vi "POLARIS Image Viewer.vi"() -> ()   [LabVIEW 2014]
uses:
  XDisplay/POLARIS IMAQ Display.xctl
  XDisplay/Properties/ImageSource.ctl
  Analyze Classes/Analyze BaseClass/Analyze BaseClass.lvclass
  Utility/POLARIS Vision utility.lvlib
panel:
  out "error out":errorcluster
  in  "File":path=path "D:/Test XDisplay images/Test TargetFocus/Test Report REad_A4 q=0,00  A=Inf µm2 _JustageCam 201410-30 16.08.30 - Kopie.png"
  out "XDisplay":cluster{"Image":T1}(xcontrol)={"Image"="remote image 000000000D10E76C"}
  in  "stop":bool=TRUE
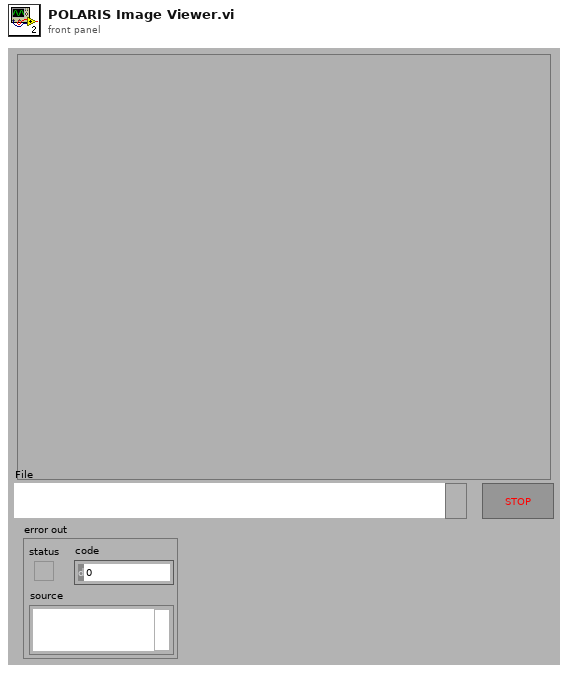
[diagram p1: front panel]
types:
  T1 = typedef "IMAQ Image.ctl" = refnum<image>
  T2 = typedef "POLARIS IMAQ Display.xctl/ImageSource.ctl" = enum16{"Camera", "File"}
  T3 = typedef "Image Type" = u32
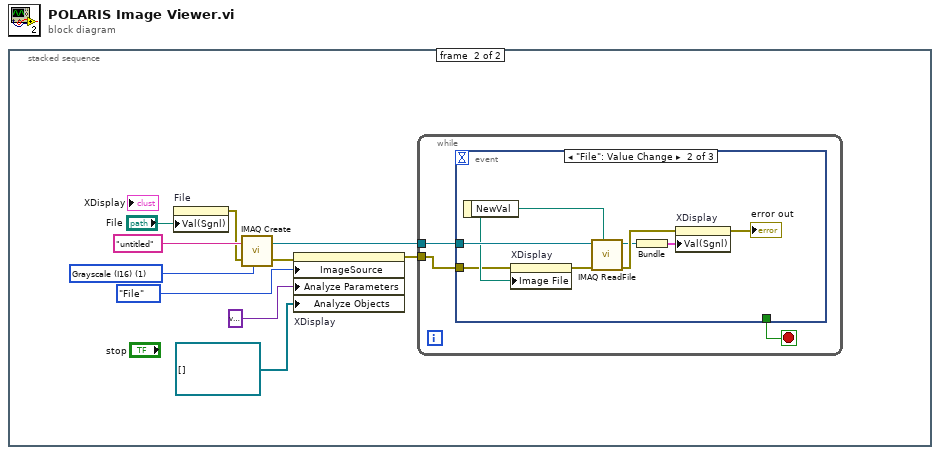
[diagram p0: block diagram]
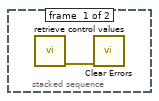
[diagram p2: hidden frame]
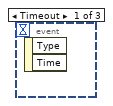
[diagram p3: hidden frame]
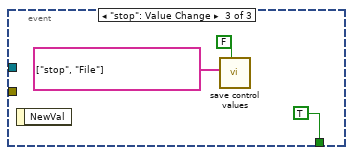
[diagram p4: hidden frame]
diagram:
  n1 = stacked-sequence {
    frame #0 {
      n2 = call "retrieve control values.vi"() -> ("error out"=w1:errorcluster)  [unwired: 10 in, 1 out]
      n3 = call <vilib>:"Clear Errors.vi"("error in (no error)"=w1) -> ()  [unwired: 5 in, 2 out]
    }
    frame #1 {
      w7 = T3 1 items=["Grayscale (U8)", "Grayscale (I16)", "Grayscale (SGL)", "Complex (CSG)", "RGB (U32)", "HSL (U32)", "RGB (U64)", "Grayscale (U16)"] ("Image Type")
      n4 = property on="File" class="Path"("Val(Sgnl)"="File") -> (error out=w4:errorcluster)  [unwired: 2 in, 1 out]
      n5 = call "IMAQ Create"("Image Name"="untitled", "Image Type"=w7, "error in (no error)"=w4) -> ("New Image"=w10:T1, "error out"=w9:errorcluster)  [unwired: 2 in]
      n6 = property on="XDisplay" class="POLARIS IMAQ Display (strict)"(error in=w9, "ImageSource"=ImageSource."File", "Analyze Parameters"=variant, "Analyze Objects"=refnum<class "Analyze BaseClass.lvclass">[] []) -> (error out=w6:errorcluster)  [unwired: 1 in, 1 out]
      n7 = while {
        tunnel: w6 -> [w12]
        tunnel: w10 -> [w13]
        stop <- w14 stop-if-true
        n8 = event shown="[1] \"File\": Value Change" {
          selector: _ -> [_ _ _]
          dyn-events: _ -> [_ _ _]
          timeout: _ -> [_ _ _]
          tunnel: [_ _ TRUE] -> w14
          tunnel: w13 -> [_ w19 _]
          tunnel: w12 -> [_ w16 _]
          event Timeout {
            n9 = event-data() -> ()  [unwired: 1 in, 2 out]
          }
          event "File": Value Change {
            n10 = event-data() -> ("NewVal"=w17:path)  [unwired: 1 in]
            n11 = property on="XDisplay" class="POLARIS IMAQ Display (strict)"(error in=w16, "Image File"=w17) -> (error out=w15:errorcluster)  [unwired: 1 in, 1 out]
            n12 = call "IMAQ ReadFile"("File Path"=w17, "error in (no error)"=w15, "Image"=w19) -> ("error out"=w21:errorcluster, "Image Out"=w20:T1)  [unwired: 4 in, 3 out]
            n13 = Bundle("Image Out"=w20) -> (w22:cluster{"Image Out":T1})  [unwired: 1 in]
            n14 = property on="XDisplay" class="POLARIS IMAQ Display (strict)"(error in=w21, "Val(Sgnl)"=w22) -> (error out=→"error out":errorcluster)  [unwired: 1 in, 1 out]
          }
          event "stop": Value Change {
            n15 = event-data() -> ()  [unwired: 1 in, 1 out]
            n16 = call "save control values.vi"("Append timestamp (true)"=FALSE, "Dont save"=string[] ["stop", "File"]) -> ()  [unwired: 6 in, 2 out]
          }
        }
      }
    }
  }
